vi "StatusOKUpdate.vi"(8 "error in (no error)":errorcluster, 10 "OkIn":bool=TRUE, 11 "Picomotor8742Comm in":refnum<class "ASCIICommClass.lvclass">) -> (0 "error out":errorcluster, 3 "Picomotor8742Comm out":refnum<class "ASCIICommClass.lvclass">)   [LabVIEW 2020, in "ASCIICommClass.lvclass"]
uses:
  ASCIICommClass.lvclass
  ASCIICommClass.lvclass/ASCIICommClass.ctl
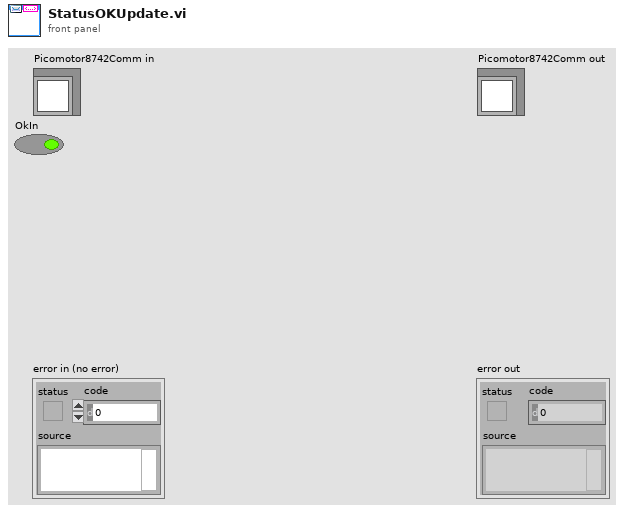
[diagram p1: front panel]
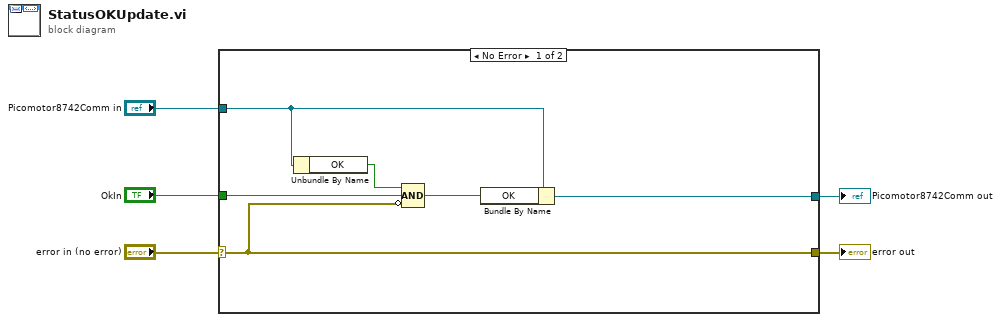
[diagram p0: block diagram]
diagram:
  n1 = case shown="No Error" "error in (no error)" {
    selector: "error in (no error)" -> [w7 w13]
    tunnel: [w7 w13] -> w4
    tunnel: [w10 w12] -> w2
    tunnel: "Picomotor8742Comm in" -> [w11 w12]
    tunnel: "OkIn" -> [w8 _]
    frame No Error {
      n2 = Unbundle By Name(w11) -> ("OK"=w6:bool)
      n3 = Compound Arithmetic op=AND(w6, w8, invert w7) -> (w9:bool)
      n4 = Bundle By Name(cluster=w11, "OK"=w9) -> (w10:refnum<class "ASCIICommClass.lvclass">)
    }
    frame Error {
    }
  }
  "error out" <- w4
  "Picomotor8742Comm out" <- w2
